vi "SetStageSpeed.vi"(8 "error in":errorcluster, 9 "Stage":T1, 10 "Z.pos":dbl, 11 "reference in":refnum<k7>) -> (0 "error out":errorcluster, 2 "result string":string, 3 "reference out":refnum<k7>)   [LabVIEW 2020]
uses:
  StageSelector--Enum.ctl
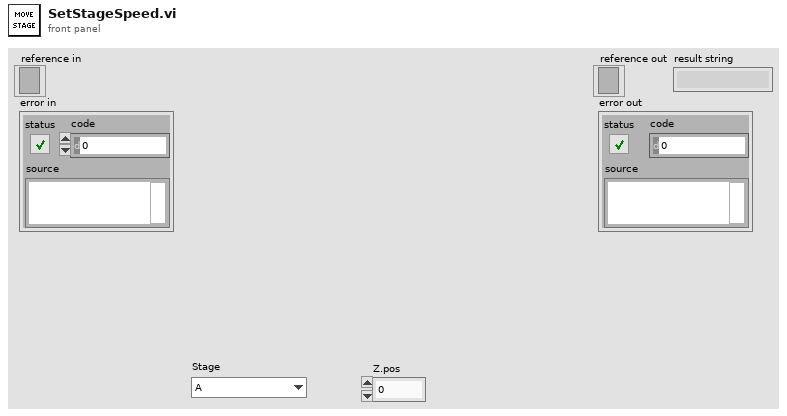
[diagram p1: front panel]
types:
  T1 = typedef "StageSelector--Enum.ctl" = enum16{"A", "B", "C", "D"}
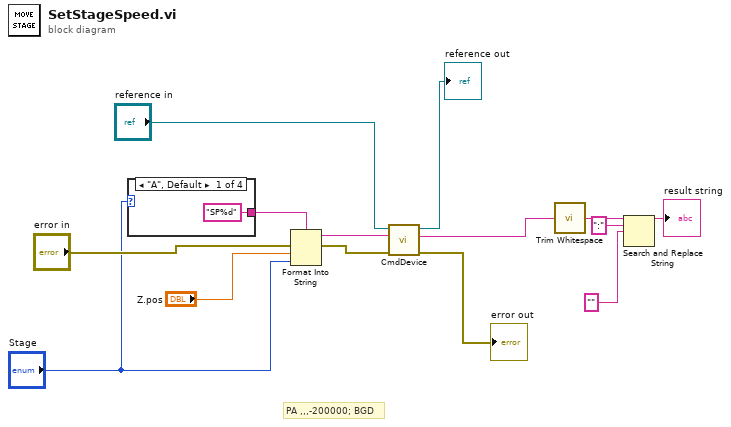
[diagram p0: block diagram]
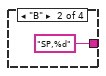
[diagram p2: hidden frame]
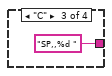
[diagram p3: hidden frame]
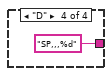
[diagram p4: hidden frame]
diagram:
  # "PA ,,,-200000; BGD"
  n1 = case shown="\"A\", Default" "Stage" {
    tunnel: ["SP%d" ("format string") "SP,%d" ("format string") "SP,,%d " ("format string") "SP,,,%d" ("format string")] -> w14
    frame "A", Default {
    }
    frame "B" {
    }
    frame "C" {
    }
    frame "D" {
    }
  }
  n2 = Format Into String(format string=w14, error in="error in", "Z.pos", "Stage") -> (resulting string=w2:string, error out=w10:errorcluster)  [unwired: 1 in]
  n3 = call "CmdDevice.vi"("error in (no error)"=w10, "Command:"=w2, "reference in"="reference in") -> ("error out"=→"error out":errorcluster, "Response:"=w4:string, "reference out"=→"reference out":refnum<k7>)  [unwired: 6 in]
  n4 = call <vilib>:"Trim Whitespace.vi"("string"=w4) -> ("trimmed string"=w7:string)  [unwired: 1 in]
  n5 = Search and Replace String(input string=w7, search string=":", replace string="" ("replace string (\"\")")) -> (result string=→"result string":string)  [unwired: 5 in, 3 out]
